vi "Query Marker.vi"(8 "error in (no error)":errorcluster, 10 "Marker Number":u8=1, 11 "VNA-ENA in":refnum<class "VNA-ENA.lvclass">) -> (0 "error out":errorcluster, 1 "Data":dbl, 2 "Frequency":dbl, 3 "VNA-ENA out":refnum<class "VNA-ENA.lvclass">)   [LabVIEW 2020, in "VNA-ENA.lvclass"]
doc: "Query the marker on the active trace"
uses:
  VNA-ENA.lvclass
  C:/Sandbox/RF Bench/Source Code/WiSpry Test Framework/Instruments/Instrument.lvclass
  Instrument.lvclass/Instrument.ctl
  Instrument.lvclass
  <instrlib>/Agilent ENA Series/Agilent ENA Series.lvlib
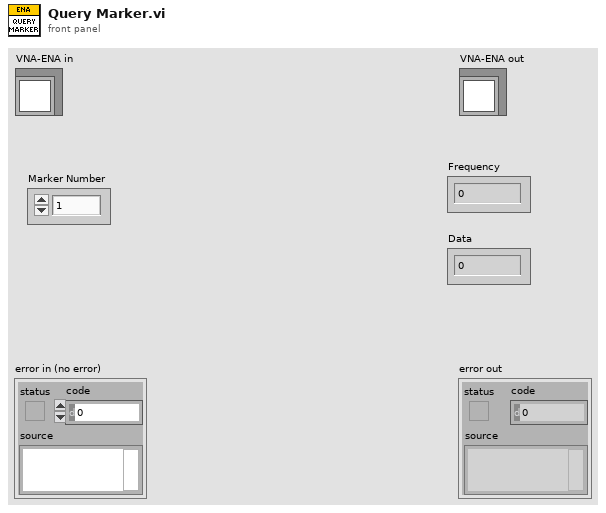
[diagram p1: front panel]
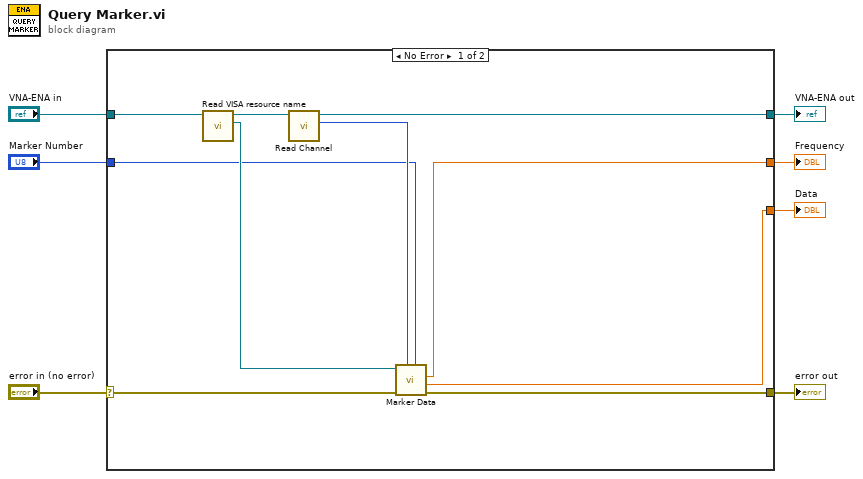
[diagram p0: block diagram]
diagram:
  n1 = case shown="No Error" "error in (no error)" {
    selector: "error in (no error)" -> [w14 w19]
    tunnel: [w13 w19] -> w7
    tunnel: [w16 w18] -> w6
    tunnel: "VNA-ENA in" -> [w17 w18]
    tunnel: "Marker Number" -> [w10 _]
    tunnel: [w9 _] -> w2
    tunnel: [w8 _] -> w1
    frame No Error {
      n2 = call "Read VISA resource name.vi"("Instrument in"=w17) -> ("VISA resource name"=w11:refnum<visa-resource-name>, "Instrument out"=w15:refnum<class "VNA-ENA.lvclass">)  [unwired: 9 in]
      n3 = call-dynamic "Read Channel.vi"("Vector Network Analyzer in"=w15) -> ("Channel"=w12:i32, "Vector Network Analyzer out"=w16:refnum<class "VNA-ENA.lvclass">)  [unwired: 9 in]
      n4 = call <instrlib>:"Marker Data.vi"("Marker (1)"=w10, "Channel (1)"=w12, "error in (no error)"=w14, "VISA resource name"=w11) -> ("error out"=w13:errorcluster, "Y Real Value"=w8:dbl, "X Value"=w9:dbl)  [unwired: 3 in, 2 out]
    }
    frame Error {
    }
  }
  "error out" <- w7
  "VNA-ENA out" <- w6
  "Data" <- w1
  "Frequency" <- w2
